vi "TDTSyn-Get Tank Codes.vi"(0 "TTankX in":refnum<k7>) -> (4 "TTankX out":refnum<k7>, 6 "Tank Codes out":string[](array[string]))   [LabVIEW 2015]
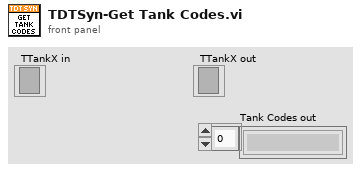
[diagram p1: front panel]
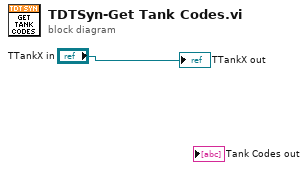
[diagram p0: block diagram]
diagram:
  "TTankX out" <- "TTankX in"
